vi "Close Log File.vi"(8 "error in (no error)":errorcluster, 11 "CSV Word Logger in":refnum<class "CSV Word Logger.lvclass">) -> (0 "error out":errorcluster, 3 "CSV Word Logger out":refnum<class "CSV Word Logger.lvclass">)   [LabVIEW 2020, in "Ballard ARINC 429 Engine.lvlib" / "Implementation.lvlib" / "CSV Word Logger.lvclass"]
uses:
  CSV Word Logger.lvclass
  CSV Word Logger.lvclass/CSV Word Logger.ctl
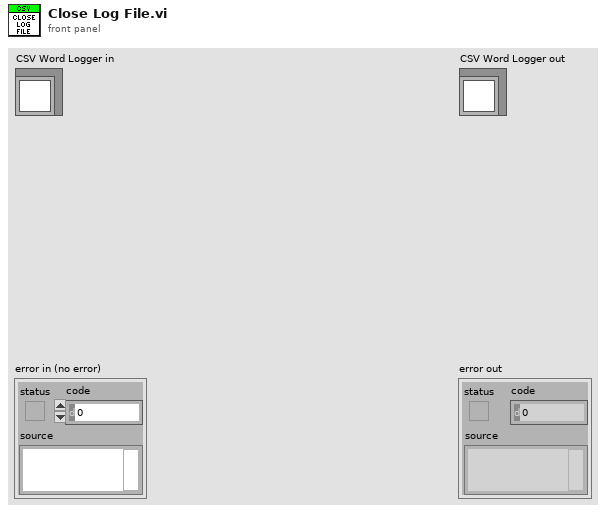
[diagram p1: front panel]
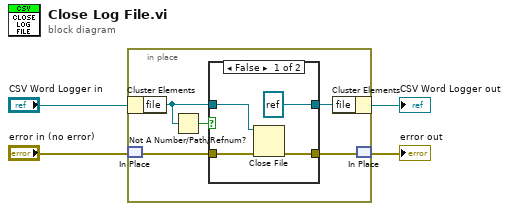
[diagram p0: block diagram]
diagram:
  n1 = in-place {
    n2 = in-place-cluster #1("CSV Word Logger in") -> ("file"=w6:refnum<file>)
    n3 = in-place-match #2("error in (no error)") -> (w8:errorcluster)
    n4 = Not A Number/Path/Refnum?(number/path/refnum=w6) -> (NaN/Path/Refnum?=w5:bool)
    n5 = case shown="False" w5 {
      tunnel: w6 -> [w13 w14]
      tunnel: [refnum<file> refnum ("file") w14] -> w9
      tunnel: w8 -> [w11 w15]
      tunnel: [w10 w15] -> w7
      frame False {
        n6 = Close File(refnum=w13, error in=w11) -> (error out=w10:errorcluster)  [unwired: 1 out]
      }
      frame True {
      }
    }
    n7 = in-place-cluster #1("file"=w9) -> (→"CSV Word Logger out":refnum<class "CSV Word Logger.lvclass">)
    n8 = in-place-match #2(w7) -> (→"error out":errorcluster)
  }
